vi "Multiple Register.vi"() -> ()   [LabVIEW 2018]
uses:
  api/Logging.lvlib
panel:
  out "multiple register test":bool
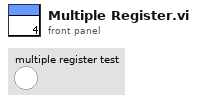
[diagram p1: front panel]
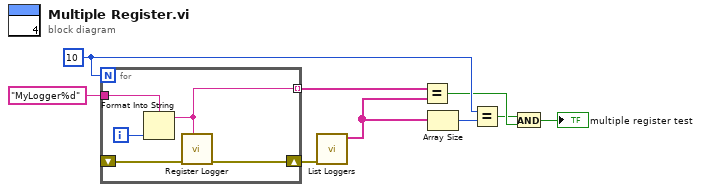
[diagram p0: block diagram]
diagram:
  w8 = 10
  n1 = for {
    N: w8 -> [_]
    tunnel: "MyLogger%d" ("name") -> [w13]
    tunnel: [w12] -> w7 mode=indexing
    shift-right: [w10] -> w1
    shift-left: _ -> [w11]
    i -> [w14]
    n2 = Format Into String(format string=w13, w14) -> (resulting string=w12:string)  [unwired: 2 in, 1 out]
    n3 = call "Register Logger.vi"("name (\"Default\")"=w12, "error in (no error)"=w11) -> ("error out"=w10:errorcluster)  [unwired: 9 in]
  }
  n4 = call "List Loggers.vi"("error in (no error)"=w1) -> ("registered loggers"=w6:string[])  [unwired: 9 in, 1 out]
  n5 = Equal?(x=w7, y=w6) -> (x = y?=w5:bool)
  n6 = Array Size(array=w6) -> (size(s)=w9:i32)
  n7 = Equal?(x=w8, y=w9) -> (x = y?=w3:bool)
  n8 = And(x=w3, y=w5) -> (x .and. y?=→"multiple register test":bool)
